vi "ServiceWaitState.vi"(8 "error in (no error)":errorcluster, 10 "Cluster in":T2, 11 "Enum in":T1) -> (0 "error out":errorcluster, 2 "Cluster out":T2, 3 "Enum":T1)   [LabVIEW 2018]
uses:
  Type_Def/Type_Def Actuator Controls.ctl
  Type_Def/Type_Def ControlState.ctl
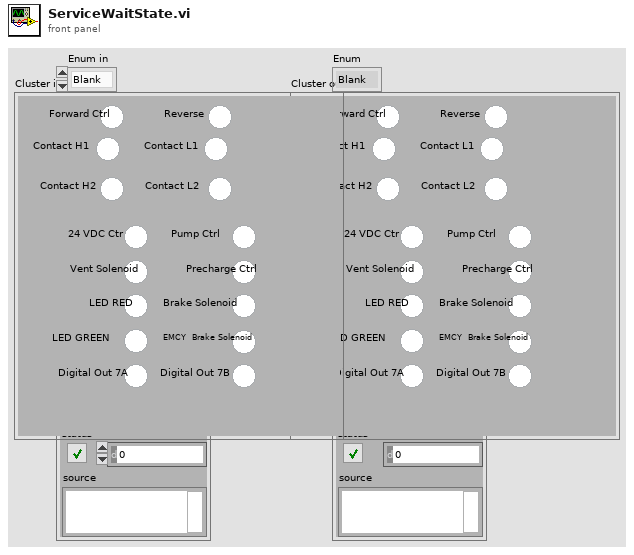
[diagram p1: front panel]
types:
  T1 = typedef "Type_Def ControlState.ctl" = enum16{"Blank", "Systems Check", "Idle", "Ready", "Pushing", "CrawlingPrecharge", "Braking", "Fault", "Boot Up", "Crawling", "Shutdown", "Service Push", "Service Wait", "Vent", "Precharge"}
  T2 = typedef "Type_Def Actuator Controls.ctl" = cluster{"Reverse ":bool, "Precharge Ctrl":bool, "Pump Ctrl":bool, "24 VDC Ctr":bool, "Vent Solenoid":bool, "Brake Solenoid":bool, "EMCY  Brake Solenoid":bool, "Digital Out 7B ":bool, "Forward Ctrl":bool, " Contact H2":bool, "Contact L2":bool, "LED RED":bool, "LED GREEN":bool, " Digital Out 7A":bool, " Contact H1":bool, "Contact L1":bool}
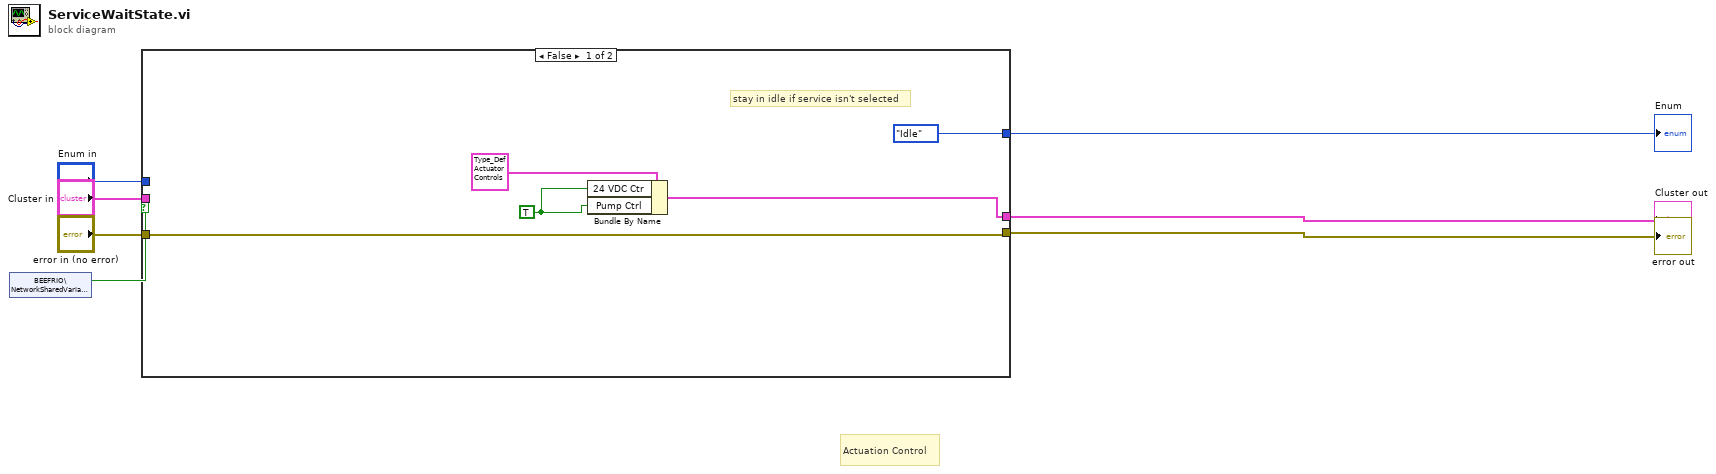
[diagram p0: block diagram]
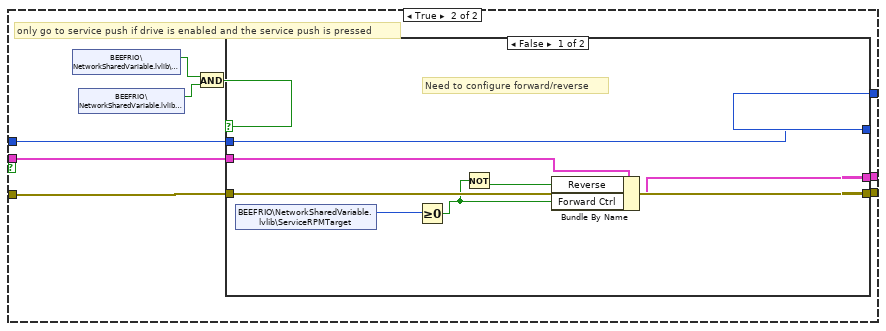
[diagram p2: hidden frame]
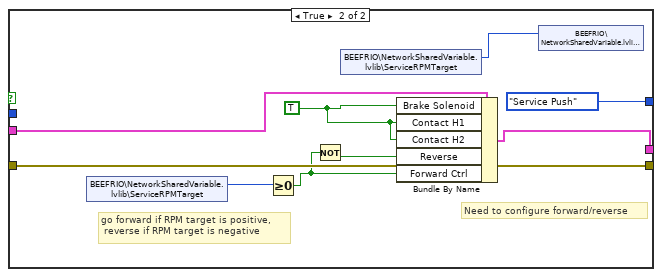
[diagram p3: hidden frame]
diagram:
  # "Actuation Control"
  n1 = shared-variable "BEEFRIO\\NetworkSharedVariable.lvlib\\Service"() -> (w1:bool)  [unwired: 1 in, 1 out]
  n2 = case shown="False" w1 {
    tunnel: "error in (no error)" -> [w12 w21]
    tunnel: [w12 w20] -> w6
    tunnel: [w9 w19] -> w5
    tunnel: "Cluster in" -> [_ w18]
    tunnel: [Type_Def_ControlState."Idle" w17] -> w3
    tunnel: "Enum in" -> [_ w16]
    frame False {
      w8 = TRUE
      # "stay in idle if service isn't selected"
      n3 = Bundle By Name(cluster=T2 {"Reverse "=FALSE, "Precharge Ctrl"=FALSE, "Pump Ctrl"=FALSE, "24 VDC Ctr"=FALSE, "Vent Solenoid"=FALSE, "Brake Solenoid"=FALSE, "EMCY  Brake Solenoid"=FALSE, "Digital Out 7B "=FALSE, "Forward Ctrl"=FALSE, " Contact H2"=FALSE, "Contact L2"=FALSE, "LED RED"=FALSE, "LED GREEN"=FALSE, " Digital Out 7A"=FALSE, " Contact H1"=FALSE, "Contact L1"=FALSE} ("Cluster in 2"), "24 VDC Ctr"=w8, "Pump Ctrl"=w8) -> (w9:T2)
    }
    frame True {
      # "only go to service push if drive is enabled and the service push is pressed"
      n4 = shared-variable "BEEFRIO\\NetworkSharedVariable.lvlib\\ServicePush"() -> (w15:bool)  [unwired: 1 in, 1 out]
      n5 = shared-variable "BEEFRIO\\NetworkSharedVariable.lvlib\\driveEnable"() -> (w13:bool)  [unwired: 1 in, 1 out]
      n6 = And(x=w15, y=w13) -> (x .and. y?=w14:bool)
      n7 = case shown="False" w14 {
        tunnel: w16 -> [w28 _]
        tunnel: [w28 Type_Def_ControlState."Service Push"] -> w17
        tunnel: w18 -> [w23 w34]
        tunnel: [w22 w35] -> w19
        tunnel: [w27 w36] -> w20
        tunnel: w21 -> [w27 w36]
        frame False {
          # "Need to configure forward/reverse"
          n8 = shared-variable "BEEFRIO\\NetworkSharedVariable.lvlib\\ServiceRPMTarget"() -> (w25:i16)  [unwired: 1 in, 1 out]
          n9 = Greater Or Equal To 0?(x=w25) -> (x >= 0?=w24:bool)
          n10 = Not(x=w24) -> (.not. x?=w26:bool)
          n11 = Bundle By Name(cluster=w23, "Reverse"=w26, "Forward Ctrl"=w24) -> (w22:T2)
        }
        frame True {
          w29 = TRUE ("Digital Out 5")
          # "go forward if RPM target is positive,\n reverse if RPM target is negative"
          # "Need to configure forward/reverse"
          n12 = shared-variable "BEEFRIO\\NetworkSharedVariable.lvlib\\ServiceRPMTarget"() -> (w31:i16)  [unwired: 1 in, 1 out]
          n13 = Greater Or Equal To 0?(x=w31) -> (x >= 0?=w30:bool)
          n14 = Not(x=w30) -> (.not. x?=w33:bool)
          n15 = shared-variable "BEEFRIO\\NetworkSharedVariable.lvlib\\ServiceRPMTarget"() -> (w32:i16)  [unwired: 1 in, 1 out]
          n16 = Bundle By Name(cluster=w34, "Brake Solenoid"=w29, "Contact H1"=w29, "Contact H2"=w29, "Reverse"=w33, "Forward Ctrl"=w30) -> (w35:T2)
          n17 = shared-variable "BEEFRIO\\NetworkSharedVariable.lvlib\\driveTarget"(w32) -> ()  [unwired: 1 in, 1 out]
        }
      }
    }
  }
  "error out" <- w6
  "Cluster out" <- w5
  "Enum" <- w3
